vi "MuC_Read_SMPL.vi"(0 "VISA resource name":refnum<visa-resource-name>, 1 "error in (no error)":errorcluster) -> (2 "VISA resource name 2":refnum<visa-resource-name>, 3 "Cmd":string, 4 "error out":errorcluster)   [LabVIEW 2019]
doc: "Send a command to a MicroController telling it to read the data in buffer. \n\nIn the case of an SMPL read the microcontroller performs single read and returns voltage at all analog input pins\n\nThe command for SMPL read as understood by the microcontroller is 's'\n\nR. Sheehan 25 - 1 - 2021"
uses:
  <vilib>/regexp/Match Regular Expression.xnode
panel:
  out "return count":u32
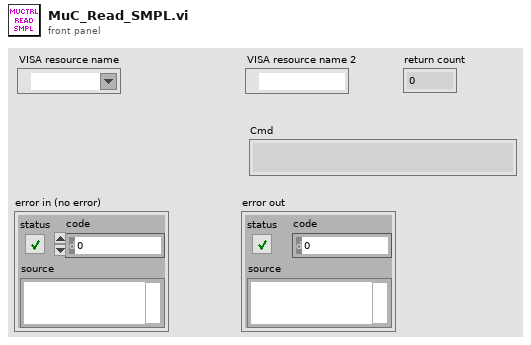
[diagram p1: front panel]
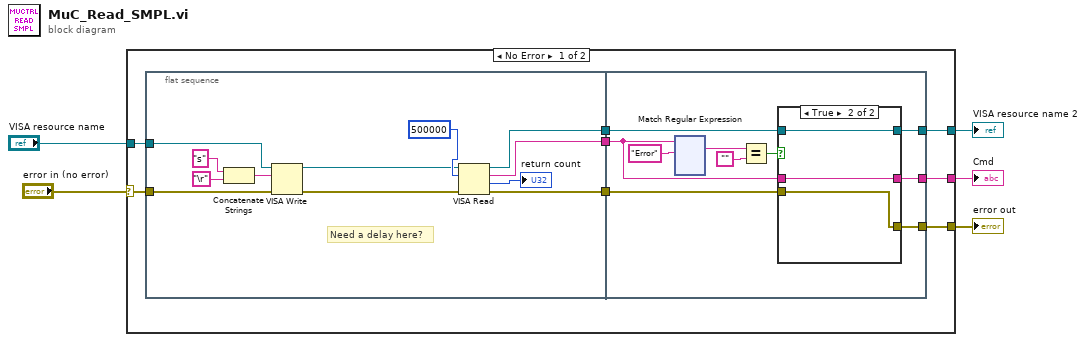
[diagram p0: block diagram]
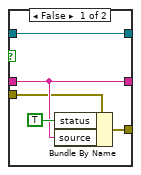
[diagram p2: hidden frame]
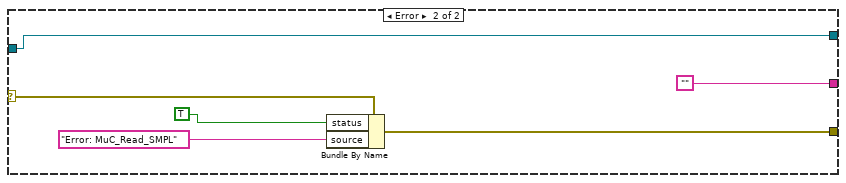
[diagram p3: hidden frame]
diagram:
  n1 = case shown="No Error" "error in (no error)" {
    selector: "error in (no error)" -> [w12 w163]
    tunnel: [w8 w162] -> w4
    tunnel: "VISA resource name" -> [w13 w159]
    tunnel: [w6 w159] -> w2
    tunnel: [w10 ""] -> w1
    frame No Error {
      n2 = flat-sequence {
        tunnel: [w17] -> w11
        tunnel: [w16] -> w9
        tunnel: [w15] -> w7
        tunnel: w13 -> [w19]
        tunnel: w12 -> [w18]
        tunnel: w11 -> [w31]
        tunnel: [w30] -> w10
        tunnel: w9 -> [w29]
        tunnel: [w28] -> w8
        tunnel: w7 -> [w27]
        tunnel: [w26] -> w6
        frame #0 {
          # "Need a delay here?"
          n3 = Concatenate Strings("s" ("string"), "\r") -> (w20:string)
          n4 = VISA Write(VISA resource name=w19, write buffer=w20, error in (no error)=w18) -> (VISA resource name out=w21:refnum<visa-resource-name>, error out=w22:errorcluster)  [unwired: 1 out]
          n5 = VISA Read(VISA resource name=w21, byte count=u32 500000, error in (no error)=w22) -> (VISA resource name out=w15:refnum<visa-resource-name>, read buffer=w17:string, return count=→"return count":u32, error out=w16:errorcluster)
        }
        frame #1 {
          n6 = xnode "Match Regular Expression"("input string"=w31, "regular expression"="Error") -> ("whole match"=w33:string)  [unwired: 4 in, 4 out]
          n7 = Equal?(x=w33, y="") -> (x = y?=w32:bool)
          n8 = case shown="True" w32 {
            tunnel: [w39 w41] -> w28
            tunnel: w31 -> [w38 w42]
            tunnel: [w38 w42] -> w30
            tunnel: w29 -> [w37 w41]
            tunnel: w27 -> [w36 w43]
            tunnel: [w36 w43] -> w26
            frame False {
              n9 = Bundle By Name(cluster=w37, "status"=TRUE, "source"=w38) -> (w39:errorcluster)
            }
            frame True {
            }
          }
        }
      }
    }
    frame Error {
      n10 = Bundle By Name(cluster=w163, "status"=TRUE, "source"="Error: MuC_Read_SMPL") -> (w162:errorcluster)
    }
  }
  "error out" <- w4
  "VISA resource name 2" <- w2
  "Cmd" <- w1
